vi "velocity-number-in-counts-per-sec-k1.vi"(9 "unit":T1(ring), 11 "velovity":dbl) -> (1 "unit":string, 3 "counts":dbl format="%#_18f")   [LabVIEW 2009]
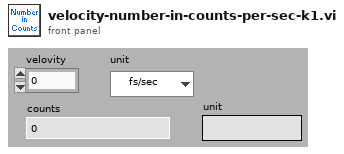
[diagram p1: front panel]
types:
  T1 = enum16{"fs/sec", "ps/sec", "um/sec", "mm/sec", "counts/sec"}
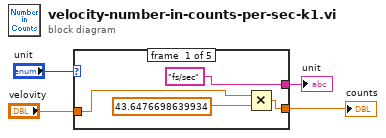
[diagram p0: block diagram]
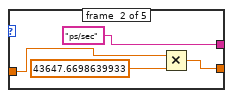
[diagram p2: hidden frame]
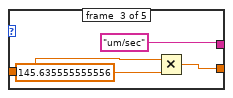
[diagram p3: hidden frame]
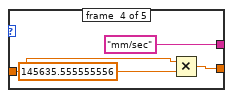
[diagram p4: hidden frame]
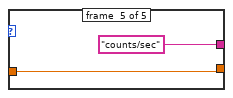
[diagram p5: hidden frame]
diagram:
  n1 = case shown="\"counts/sec\", Default" "unit" {
    tunnel: "velovity" -> [w6 w10 w14 w18 w22]
    tunnel: [w8 w12 w16 w20 w22] -> w2
    tunnel: ["fs/sec" "ps/sec" "um/sec" "mm/sec" "counts/sec"] -> w1
    frame #0 {
      n2 = Multiply(x=w6, y=43.6476698639934) -> (x*y=w8:dbl)
    }
    frame #1 {
      n3 = Multiply(x=w10, y=43647.6698639933) -> (x*y=w12:dbl)
    }
    frame #2 {
      n4 = Multiply(x=w14, y=145.635555555556) -> (x*y=w16:dbl)
    }
    frame #3 {
      n5 = Multiply(x=w18, y=145635.555555556) -> (x*y=w20:dbl)
    }
    frame #4 {
    }
  }
  "counts" <- w2
  "unit" <- w1
